vi "Listen Robot Socket.vi"() -> ()   [LabVIEW 2018]
panel:
  out "length":i32
  in  "Send Data?":bool
  in  "Stop Button":bool
  out "remote address":string="192.168.0.10"
  out "data out":string
  in  "Client Closed":string="The client VI closed the connection."
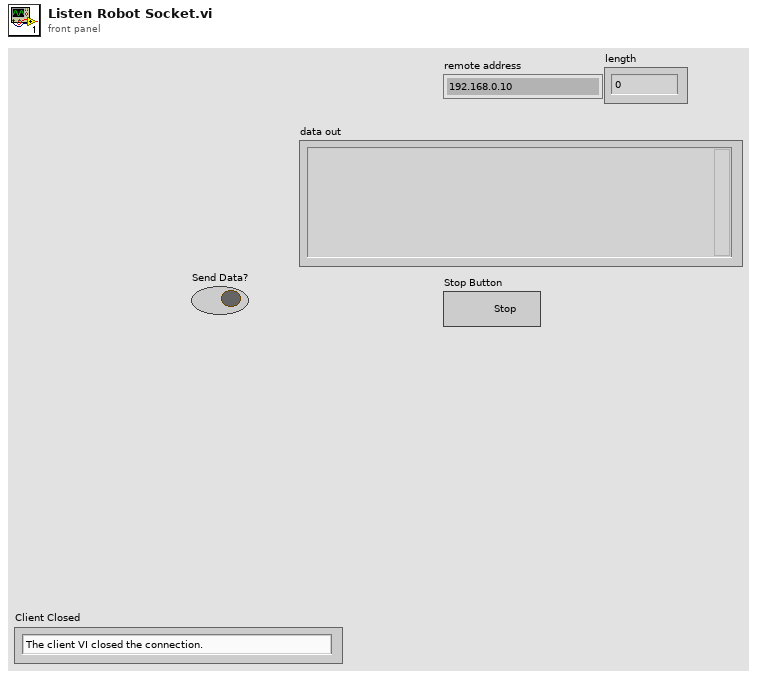
[diagram p1: front panel]
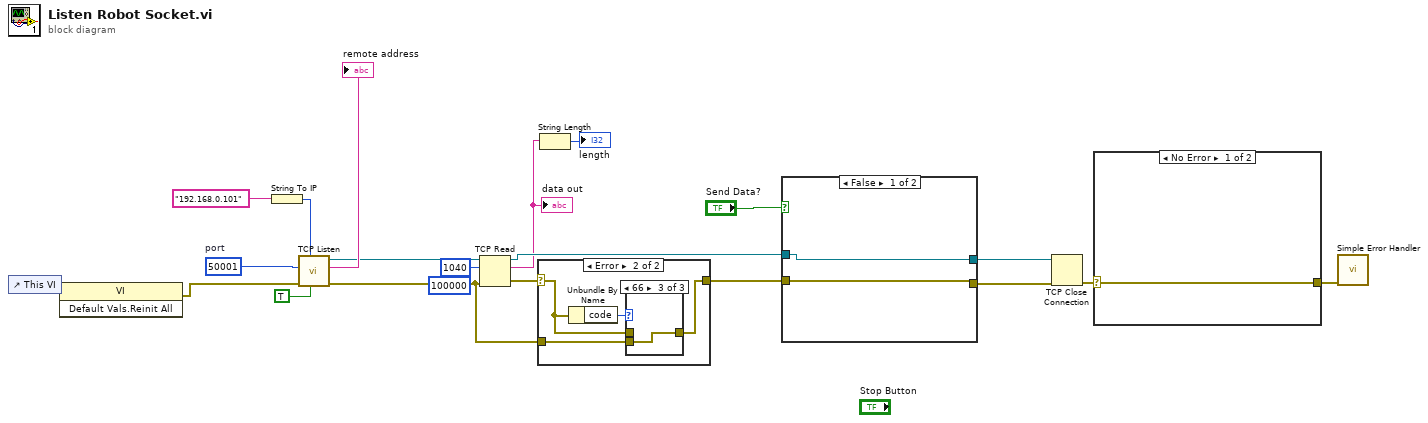
[diagram p0: block diagram]
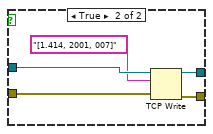
[diagram p2: hidden frame]
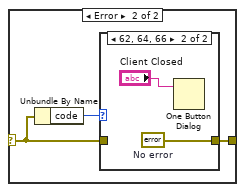
[diagram p6: hidden frame]
diagram:
  w21 = u16 50001  # port
  n1 = control-ref of="This VI"() -> (w4:refnum<vi>)
  n2 = invoke class="VI" method="Default Vals.Reinit All"(reference=w4) -> (error out=w3:errorcluster)  [unwired: 2 in, 2 out]
  n3 = String To IP(1:"192.168.0.101") -> (0:w16:u32)
  n4 = call <vilib>:"TCP Listen.vi"("resolve remote address (T)"=TRUE, "net address"=w16, "error in (no error)"=w3, "port"=w21) -> ("error out"=w20:errorcluster, "remote address"=→"remote address":string, "connection ID"=w13:refnum<k5>)  [unwired: 3 in, 2 out]
  n5 = TCP Read(connection ID=w13, bytes to read=1040, error in (no error)=w20, 9:100000 ("timeout ms (25000)")) -> (connection ID out=w9:refnum<k5>, data out=w6:string, error out=w10:errorcluster)  [unwired: 1 out]
  "data out" <- w6
  n6 = case shown="Error" w10 {
    selector: w10 -> [w22 w25]
    tunnel: [w22 w23] -> w8
    tunnel: w20 -> [_ w24]
    frame No Error {
    }
    frame Error {
      n7 = Unbundle By Name(w25) -> ("code"=w26:i32)
      n8 = case shown="66" w26 {
        tunnel: w25 -> [w27 _ _]
        tunnel: w24 -> [_ w28 w29]
        tunnel: [w27 w28 w29] -> w23
        frame Default {
        }
        frame 56 {
        }
        frame 66 {
        }
      }
    }
  }
  n9 = String Length(string=w6) -> (length=→"length":i32)
  n10 = case shown="False" "Send Data?" {
    tunnel: w9 -> [w31 w36]
    tunnel: [w31 w35] -> w12
    tunnel: w8 -> [w30 w34]
    tunnel: [w30 w33] -> w11
    frame False {
    }
    frame True {
      n11 = TCP Write(connection ID=w36, data in="[1.414, 2001, 007]", error in (no error)=w34) -> (connection ID out=w35:refnum<k5>, error out=w33:errorcluster)  [unwired: 1 in, 1 out]
    }
  }
  n12 = TCP Close Connection(connection ID=w12, error in (no error)=w11) -> (error out=w18:errorcluster)  [unwired: 2 out]
  n13 = case shown="No Error" w18 {
    selector: w18 -> [w37 w39]
    tunnel: [w37 w38] -> w19
    frame No Error {
    }
    frame Error {
      n14 = Unbundle By Name(w39) -> ("code"=w40:i32)
      n15 = case shown="62, 64, 66" w40 {
        tunnel: w39 -> [w41 _]
        tunnel: [w41 w43] -> w38
        frame Default {
        }
        frame 62, 64, 66 {
          w43 = errorcluster {"status"=FALSE, "code"=0, "source"=""}  # No error
          n16 = One Button Dialog(message="Client Closed") -> ()  [unwired: 1 in, 1 out]
        }
      }
    }
  }
  n17 = call <vilib>:"Simple Error Handler.vi"("error in (no error)"=w19) -> ()  [unwired: 1 in, 8 out]
